vi "Set Mode.vi"(8 "error in (no error)":errorcluster, 10 "Mode":T1=enum."Run", 11 "Cfg Grandmaster in":refnum<class "Cfg Grandmaster.lvclass">) -> (0 "error out":errorcluster, 3 "Cfg Grandmaster out":refnum<class "Cfg Grandmaster.lvclass">)   [LabVIEW 2012, in "Configuration Grandmaster.lvlib" / "Cfg Grandmaster.lvclass"]
uses:
  Cfg Grandmaster.lvclass
  Common/Controls/DAQMan Mode.ctl
  Cfg Grandmaster.lvclass/Cfg Grandmaster.ctl
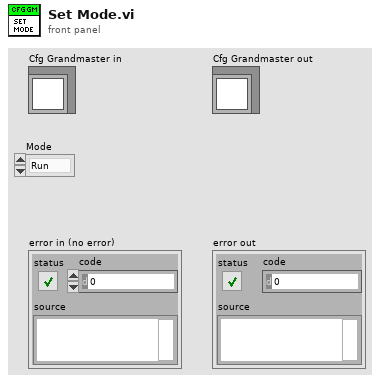
[diagram p1: front panel]
types:
  T1 = typedef "DAQMan Mode.ctl" = enum16{"Cfg", "Run", "Shutting Down"}
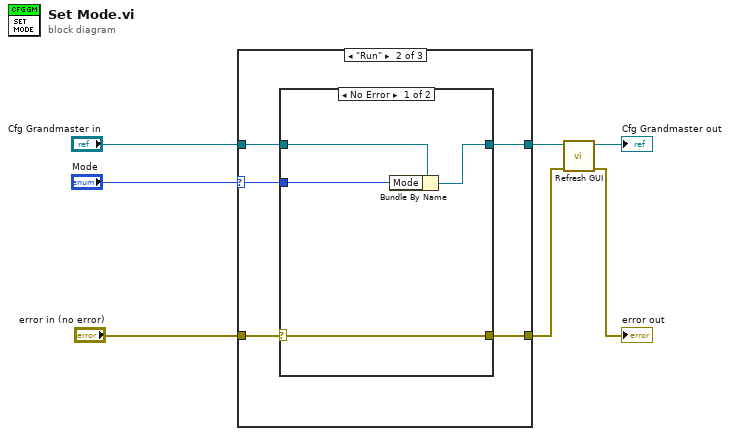
[diagram p0: block diagram]
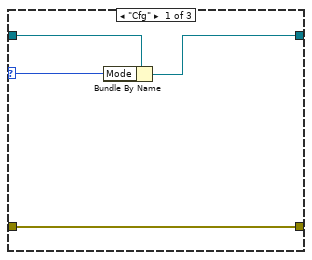
[diagram p2: hidden frame]
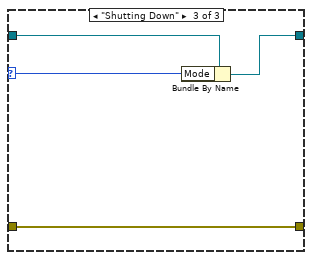
[diagram p4: hidden frame]
diagram:
  n1 = case shown="\"Run\"" "Mode" {
    selector: "Mode" -> [w9 w13 w26]
    tunnel: [w10 w16 w24] -> w4
    tunnel: "Cfg Grandmaster in" -> [w11 w15 w25]
    tunnel: "error in (no error)" -> [w8 w14 w23]
    tunnel: [w8 w12 w23] -> w2
    frame "Cfg" {
      n2 = Bundle By Name(cluster=w11, "Mode"=w9) -> (w10:refnum<class "Cfg Grandmaster.lvclass">)
    }
    frame "Run" {
      n3 = case shown="No Error" w14 {
        selector: w14 -> [w17 w22]
        tunnel: [w17 w22] -> w12
        tunnel: w15 -> [w20 w21]
        tunnel: [w19 w21] -> w16
        tunnel: w13 -> [w18 _]
        frame No Error {
          n4 = Bundle By Name(cluster=w20, "Mode"=w18) -> (w19:refnum<class "Cfg Grandmaster.lvclass">)
        }
        frame Error {
        }
      }
    }
    frame "Shutting Down" {
      n5 = Bundle By Name(cluster=w25, "Mode"=w26) -> (w24:refnum<class "Cfg Grandmaster.lvclass">)
    }
  }
  n6 = call "Refresh GUI.vi"("error in (no error)"=w2, "Cfg Grandmaster in"=w4) -> ("error out"=→"error out":errorcluster, "Cfg Grandmaster out"=→"Cfg Grandmaster out":refnum<class "Cfg Grandmaster.lvclass">)  [unwired: 8 in]
